vi "Comprobación Señal digital (SubVI).vi"(1 "Inductivo":sgl[](array[numeric])) -> (0 "Señal digital?":bool)   [LabVIEW 2015]
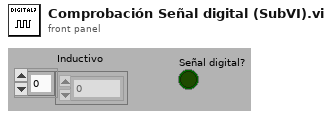
[diagram p1: front panel]
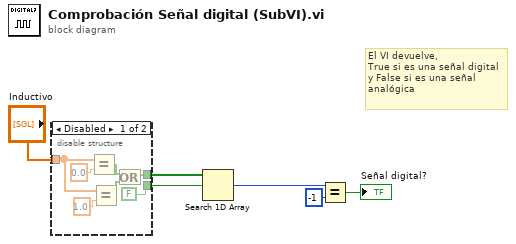
[diagram p0: block diagram]
diagram:
  # "El VI devuelve,\nTrue si es una señal digital\ny False si es una señal\nanalógica"
  n1 = disable-structure shown="Disabled" {
    disable-tunnel: [FALSE ("element") _] -> w3
    disable-tunnel: [w12 _] -> w2
    disable-tunnel: "Inductivo" -> [w9 _]
    frame Disabled {
      n2 = Equal?(x=w9, y=0.0) -> (x = y?=w10:bool[])
      n3 = Equal?(x=w9, y=1.0) -> (x = y?=w11:bool[])
      n4 = Or(x=w10, y=w11) -> (x .or. y?=w12:bool[])
    }
    frame Enabled {
    }
  }
  n5 = Search 1D Array(1D array=w2, element=w3) -> (index of element=w4:i32)  [unwired: 1 in]
  n6 = Equal?(x=w4, y=-1) -> (x = y?=→"Señal digital?":bool)
